vi "Load Sequence HTTP.vi"(8 "error in (no error)":errorcluster, 9 "VSEQ":string="{\n    \"Sequence\": {\n        \"Name\": \"Bottle Condition\",\n        \"Version\": \"1\",\n        \"Comment\": \"Control state machine for bottle heating/cooling.\",\n        \"Entry\": \"Start\",\n        \"Abort\": \"Stop\",\n        \"States\": {\n            \"Start\": {\n                \"Comment\": \"Reset bottle controls to off state.\",\n                \"Steps\": [\n                    {\n                        \"Time\": 0,\n                        \"Commands\": [\n                            {\"Type\": \"Transition\", \"Target\": \"Hold\"}\n                        ]\n                    }\n                ]\n            },\n            \"Hold\": {\n                \"Comment\": \"Bottle in range, controls off.\",\n                \"Steps\": [\n                    {\n                        \"Time\": 0,\n                        \"Commands\": [\n                            {\"Type\": \"Digital\", \"Channel\": \"BottleCool\", \"Value\": false},\n                            {\"Type\": \"Digital\", \"Channel\": \"BottleHeat\", \"Value\": false}\n                        ]\n                    }\n                ],\n                \"Transitions\": [\n                    {\n                        \"Type\": \"State\",\n                        \"Target\": \"Cool\",\n                        \"Logic\": \"Any\",\n                        \"Conditions\": [\n                            {\"Type\": \"HighLimit\", \"Channel\": \"BottlePSI\", \"Limit\": 850}\n                        ]\n                    },\n                    {\n                        \"Type\": \"State\",\n                        \"Target\": \"Heat\",\n                        \"Logic\": \"Any\",\n                        \"Conditions\": [\n                            {\"Type\": \"LowLimit\", \"Channel\": \"BottlePSI\", \"Limit\": 750}\n                        ]\n                    }\n                ]\n            },\n            \"Cool\": {\n                \"Comment\": \"Cooling, wait for pressure to drop.\",\n                \"Steps\": [\n                    {\n                        \"Time\": 0,\n                        \"Commands\": [\n                            {\"Type\": \"Digital\", \"Channel\": \"BottleCool\", \"Value\": true}\n                        ]\n                    }\n                ],\n                \"Transitions\": [\n                    {\n                        \"Type\": \"State\",\n                        \"Target\": \"Start\",\n                        \"Logic\": \"Any\",\n                        \"Conditions\": [\n                            {\"Type\": \"LowLimit\", \"Channel\": \"BottlePSI\", \"Limit\": 800}\n                        ]\n                    }\n                ]\n            },\n            \"Heat\": {\n                \"Comment\": \"Heating, wait for pressure to rise.\",\n                \"Steps\": [\n                    {\n                        \"Time\": 0,\n                        \"Commands\": [\n                            {\"Type\": \"Digital\", \"Channel\": \"BottleHeat\", \"Value\": true}\n                        ]\n                    }\n                ],\n                \"Transitions\": [\n                    {\n                        \"Type\": \"State\",\n                        \"Target\": \"Start\",\n                        \"Logic\": \"Any\",\n                        \"Conditions\": [\n                            {\"Type\": \"HighLimit\", \"Channel\": \"BottlePSI\", \"Limit\": 800}\n                        ]\n                    }\n                ]\n            },\n            \"Stop\": {\n                \"Comment\": \"Stopping, ensure controls off.\",\n                \"Steps\": [\n                    {\n                        \"Time\": 0,\n                        \"Commands\": [\n                            {\"Type\": \"Digital\", \"Channel\": \"BottleCool\", \"Value\": false},\n                            {\"Type\": \"Digital\", \"Channel\": \"BottleHeat\", \"Value\": false},\n                            {\"Type\": \"Stop\"}\n                        ]\n                    }\n                ]\n            }\n        }\n    }\n}", 10 "URL":string="http://localhost:13083", 11 "Path":path) -> (0 "error out":errorcluster, 1 "Message":string, 2 "Success":bool)   [LabVIEW 2023, in "VolatusSeqGUI.lvlib" / "Sequencing Control.lvclass"]
uses:
  Sequencing Control.lvclass
  lv-web-crypto/lv-crypto/Crypto/Hashes/SHA-256/SHA-256.lvclass
  <vilib>/httpClient/MultipartData.ctl
  Sequencing Control.lvclass/Sequencing Control.ctl
  lv-web-crypto/lv-crypto/Crypto/Crypto.lvlib
  <vilib>/httpClient/LabVIEWHTTPClient.lvlib
  VolatusSeqConfig/Sequence Config/Sequence Config.lvclass
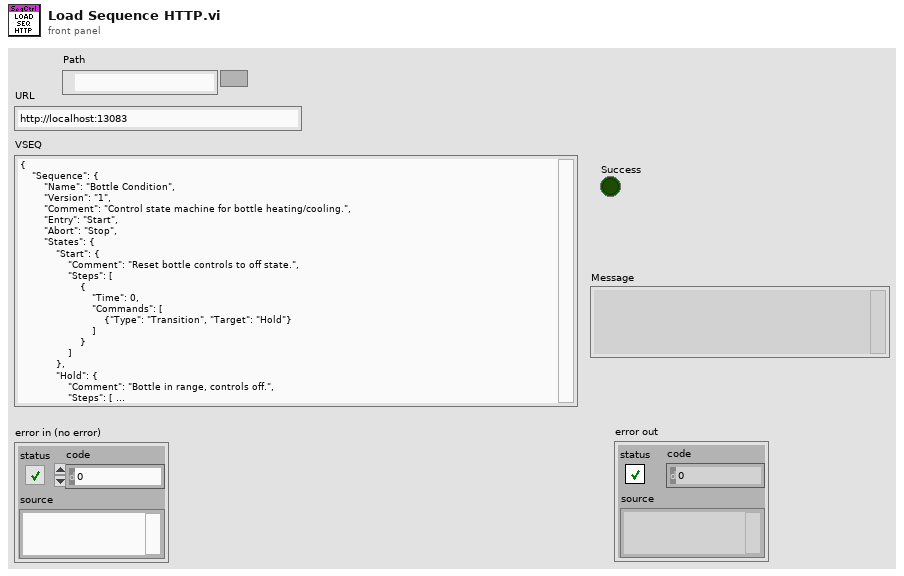
[diagram p1: front panel]
types:
  T1 = typedef "LabVIEWHTTPClient.lvlib/MultipartData.ctl" = cluster{"Name":string, "Value":string, "File":path, "Filename":string, "MIME type":string}
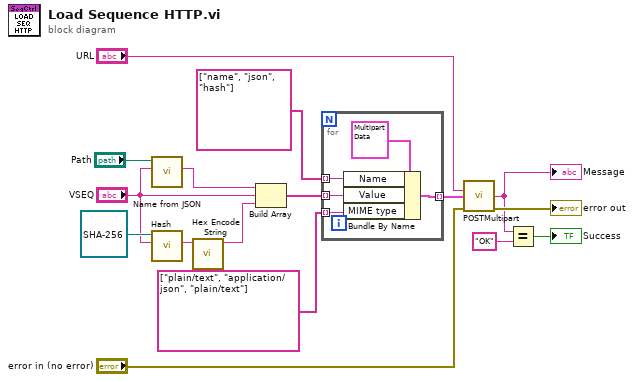
[diagram p0: block diagram]
diagram:
  n1 = call "Name from JSON.vi"("JSON"="VSEQ", "Path"="Path") -> ("Name"=w2:string)  [unwired: 8 in, 1 out]
  n2 = call-dynamic "Hash.vi"("Message"="VSEQ", "SHA-256 in"=refnum<class "SHA-256.lvclass"> refnum) -> ("Hash"=w15:string)  [unwired: 7 in, 2 out]
  n3 = call "Hex Encode String.vi"("String"=w15) -> ("Hex Encoded String"=w13:string)  [unwired: 10 in]
  n4 = Build Array(w2, "VSEQ", w13) -> (w12:string[])
  n5 = for {
    tunnel: w12 -> [w20] mode=indexing
    tunnel: string[] ["name", "json", "hash"] -> [w19] mode=indexing
    tunnel: string[] ["plain/text", "application/json", "plain/text"] -> [w18] mode=indexing
    tunnel: [w17] -> w9 mode=indexing
    n6 = Bundle By Name(cluster=T1 {"Name"="", "Value"="", "File"=path "", "Filename"="", "MIME type"="application/octet-stream"} ("Element"), "Name"=w19, "Value"=w20, "MIME type"=w18) -> (w17:T1)
  }
  n7 = call <vilib>:"POSTMultipart.vi"("url"="URL", "data"=w9, "error in (no error)"="error in (no error)") -> ("body"=w8:string, "error out"=→"error out":errorcluster)  [unwired: 9 in, 2 out]
  "Message" <- w8
  n8 = Equal?(x=w8, y="OK") -> (x = y?=→"Success":bool)
